vi "UDP Data Link - Driver Utilities - Clear Specific Error.vi"(5 "Error to Clear":i32, 6 "Error In":errorcluster) -> (0 "Error Out":errorcluster, 1 "Error Matched?":bool)   [LabVIEW 2012, in "UDP Data Link Engine.lvlib"]
doc: "Clears the specified error that you wire to the Error to Clear input. If you do not match the specific error to clear, the VI passes the original error back out."
uses:
  UDP Data Link Engine.lvlib
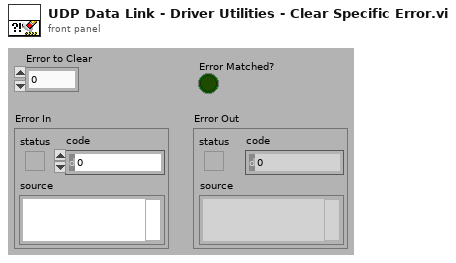
[diagram p1: front panel]
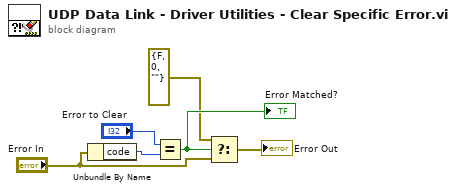
[diagram p0: block diagram]
diagram:
  n1 = Unbundle By Name("Error In") -> ("code"=w6:i32)
  n2 = Equal?(x="Error to Clear", y=w6) -> (x = y?=w3:bool)
  "Error Matched?" <- w3
  n3 = Select(t=errorcluster {"status"=FALSE, "code"=0, "source"=""}, s=w3, f="Error In") -> (s? t:f=→"Error Out":errorcluster)
